vi "Find Target.vi"(8 "error in (no error)":errorcluster, 10 "Target":string, 11 "Project in":refnum<vi>) -> (0 "error out":errorcluster, 1 "Target":refnum<vi>, 2 "TargetAppContext":refnum<vi>, 3 "Project":refnum<vi>)   [LabVIEW 2020, in "VolatusBuild.lvlib"]
uses:
  VolatusBuild.lvlib
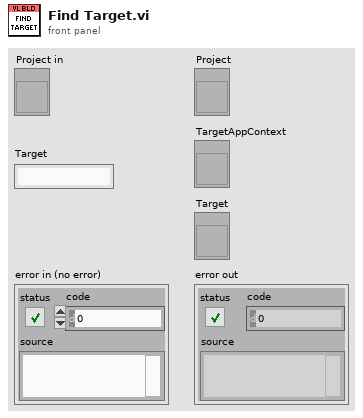
[diagram p1: front panel]
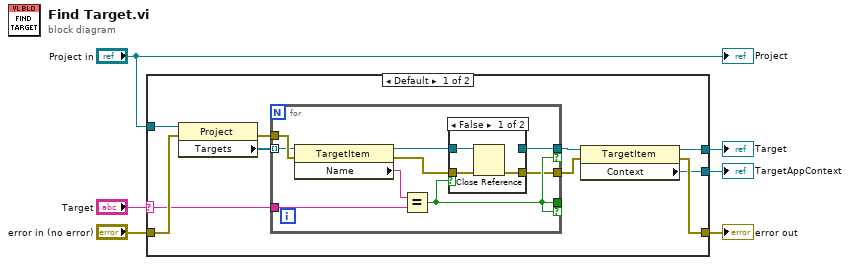
[diagram p0: block diagram]
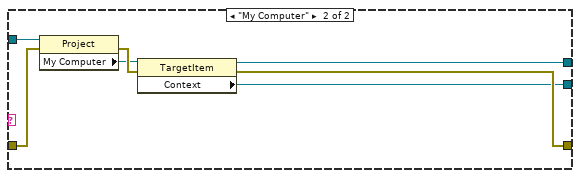
[diagram p3: hidden frame]
diagram:
  n1 = case shown="Default" "Target" {
    selector: "Target" -> [w12 _]
    tunnel: "Project in" -> [w14 w35]
    tunnel: "error in (no error)" -> [w15 w33]
    tunnel: [w9 w32] -> w4
    tunnel: [w8 w31] -> w3
    tunnel: [w16 w37] -> w2
    frame Default {
      n2 = property class="Project"(reference=w14, error in=w15) -> (error out=w11:errorcluster, "Targets"=w13:refnum<vi>[])  [unwired: 1 out]
      n3 = for {
        tunnel: w13 -> [w24] mode=indexing
        tunnel: w12 -> [w23]
        tunnel: [w19] -> _ if=w19
        tunnel: w11 -> [w25]
        tunnel: [w20] -> w10 if=w19
        tunnel: [w17] -> w7
        n4 = property class="TargetItem"(reference=w24, error in=w25) -> (reference out=w21:refnum<vi>, error out=w18:errorcluster, "Name"=w22:string)
        n5 = Equal?(x=w22, y=w23) -> (x = y?=w19:bool)
        n6 = case shown="False" w19 {
          tunnel: w21 -> [w28 w30]
          tunnel: [_ w30] -> w20
          tunnel: w18 -> [w27 w29]
          tunnel: [w26 w29] -> w17
          frame False {
            n7 = Close Reference(reference=w28, error in (no error)=w27) -> (error out=w26:errorcluster)
          }
          frame True {
          }
        }
      }
      n8 = property class="TargetItem"(reference=w10, error in=w7) -> (reference out=w9:refnum<vi>, error out=w16:errorcluster, "Context"=w8:refnum<vi>)
    }
    frame "My Computer" {
      n9 = property class="Project"(reference=w35, error in=w33) -> (error out=w36:errorcluster, "My Computer"=w34:refnum<vi>)  [unwired: 1 out]
      n10 = property class="TargetItem"(reference=w34, error in=w36) -> (reference out=w32:refnum<vi>, error out=w37:errorcluster, "Context"=w31:refnum<vi>)
    }
  }
  "error out" <- w2
  "Target" <- w4
  "TargetAppContext" <- w3
  "Project" <- "Project in"
